vi "Auto Threshold.vi"(1 "x[n]":dbl[](array[numeric]) format="%.2f") -> (0 "threshold":dbl format="%.2f")   [LabVIEW 2017, in "SoundVib_TachProcess.lvlib"]
doc: "Returns a suggested threshold for <B>x[n]</B>. Use <B>threshold</B> for pulse-edge detection."
uses:
  <vilib>/addons/Sound and Vibration/Order Analysis/Tach Process/SoundVib_TachProcess.lvlib
  <vilib>/Analysis/NI_AALBase.lvlib
panel:
  # "Auto Threshold"
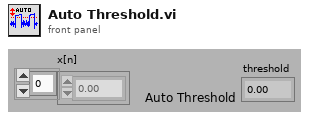
[diagram p1: front panel]
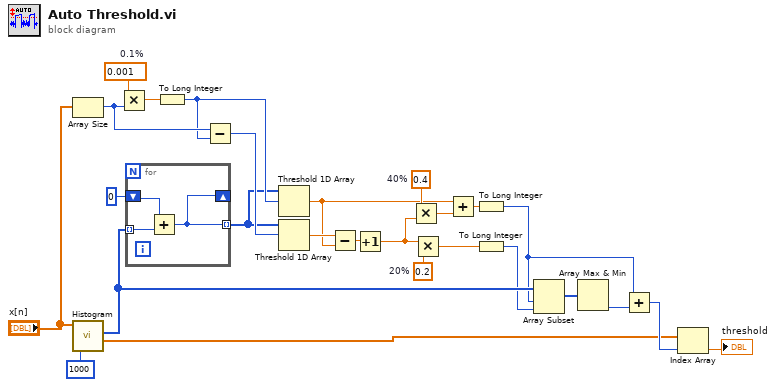
[diagram p0: block diagram]
diagram:
  w5 = 0.2  # 20%
  w9 = 0.4  # 40%
  w25 = 0.001  # 0.1%
  n1 = Array Size(array="x[n]") -> (size(s)=w22:i32)
  n2 = call <vilib>:"Histogram.vi"("intervals"=1000, "X"="x[n]") -> ("X Values"=w12:dbl[], "Histogram: h(x)"=w17:i32[])  [unwired: 6 in, 2 out]
  n3 = Multiply(x=w25, y=w22) -> (x*y=w26:dbl)
  n4 = for {
    shift-right: [w27] -> _
    shift-left: 0 -> [w28]
    tunnel: w17 -> [w29] mode=indexing
    tunnel: [w27] -> w19 mode=indexing
    n5 = Add(x=w28, y=w29) -> (x+y=w27:i32)
  }
  n6 = To Long Integer(number=w26) -> (32bit integer=w21:i32)
  n7 = Subtract(x=w22, y=w21) -> (x-y=w20:i32)
  n8 = Threshold 1D Array(2:w21, 3:w19) -> (0:w7:dbl)  [unwired: 1 in]
  n9 = Threshold 1D Array(2:w20, 3:w19) -> (0:w10:dbl)  [unwired: 1 in]
  n10 = Subtract(x=w10, y=w7) -> (x-y=w16:dbl)
  n11 = Increment(x=w16) -> (x+1=w6:dbl)
  n12 = Multiply(x=w9, y=w6) -> (x*y=w8:dbl)
  n13 = Multiply(x=w6, y=w5) -> (x*y=w3:dbl)
  n14 = Add(x=w7, y=w8) -> (x+y=w4:dbl)
  n15 = To Long Integer(number=w4) -> (32bit integer=w2:i32)
  n16 = To Long Integer(number=w3) -> (32bit integer=w1:i32)
  n17 = Array Subset(array=w17, index=w2, length=w1) -> (w15:i32[])
  n18 = Array Max & Min(array=w15) -> (min index (indices)=w14:i32)  [unwired: 3 out]
  n19 = Add(x=w2, y=w14) -> (x+y=w13:i32)
  n20 = Index Array(array=w12, index=w13) -> (element=→"threshold":dbl)
